vi "InitializeOCUCommunication.vi"(2 "error in (no error)":errorcluster) -> (0 "error out":errorcluster, 1 "NetworkStreamWriter out":refnum<class "NetworkStreamReader.lvclass">)   [LabVIEW 2013]
doc: "Initializes stream for communication with the OCU\n\nAuthored: Victoria Coleman 03/28/14"
uses:
  RIO-OCU_Comm/NetworkStreams/Reader/NetworkStreamReader.lvclass
  OCU/Location of Think.ctl
  RIO-OCU_Comm/ToRIO.ctl
  OCU/CommandMessages.ctl
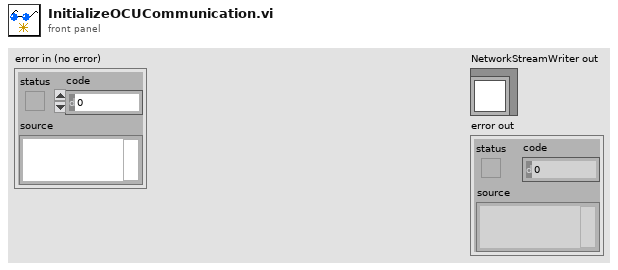
[diagram p1: front panel]
types:
  T1 = typedef "ToRIO.ctl" = cluster{"Commands":T2, "Variant":variant}
  T2 = typedef "CommandMessages.ctl" = enum16{"Pass", "OverrideMode", "Add mission", "Delete mission", "Change constants"}
  T3 = typedef "Location of Think.ctl" = string
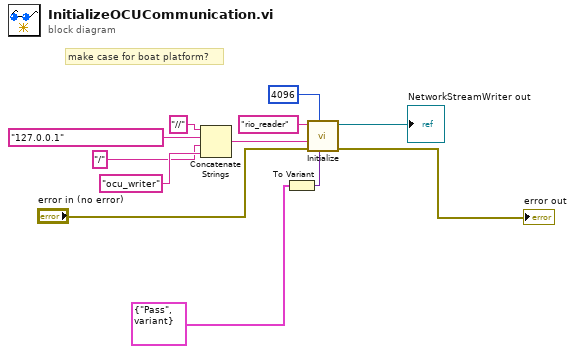
[diagram p0: block diagram]
diagram:
  # "make case for boat platform?"
  n1 = Concatenate Strings("//" ("string"), T3 "127.0.0.1" ("Location of THINK"), "/", "ocu_writer" ("string")) -> (w7:string)
  n2 = To Variant(anything=T1 {"Commands"=enum."Pass", "Variant"=variant} ("To RIO")) -> (Variant=w11:variant)
  n3 = call "Initialize.vi"("Default return"=w11, "reader buffer size"=4096 ("writer buffer size"), "error in (no error)"="error in (no error)", "writer url"=w7, "reader name"="rio_reader" ("writer name")) -> ("error out"=→"error out":errorcluster, "NetworkStreamWriter out"=→"NetworkStreamWriter out":refnum<class "NetworkStreamReader.lvclass">)  [unwired: 5 in]
